vi "DAQ setting.vi"(8 "error in (no error)":errorcluster={"status"=TRUE, "code"=1026, "source"="Invoke Node in General Config.vi->Main Window.vi"}, 11 "vi reference":refnum<vi>) -> (0 "error Out":errorcluster={"status"=TRUE, "code"=1026, "source"="Invoke Node in General Config.vi->Main Window.vi"}, 3 "Out reference":refnum<vi>)   [LabVIEW 2015]
uses:
  Control Button/Exit.ctl
  Control Button/Save.ctl
  <vilib>/addons/database/Connection.llb/DB Tools Open Connec (String).vi
  <vilib>/addons/database/_DB Variant To Data/Database Variant To Data.xnode
  <vilib>/addons/database/NI_Database_API.lvlib
panel:
  out "error out":errorcluster={"status"=TRUE, "code"=97, "source"="NI_Database_API.lvlib:DB Tools Close Connection.vi->DAQ setting.vi<ERR>ADO Error: 0x00000061\r\nUnknown System Error in NI_Database_API.lvlib:DB Tools Close Connection.vi->DAQ setting.vi"}
  in  "read":bool=TRUE
  out "subarray":string[](array[string])=["PART CLAMPING CYL-1&2 SOL(P0.17)", "PART DECLAMPING CYL-1&2 SOL (P0.18)", "FLAP LOCKING CYL FDW SOL(P0.19)", "SCREWING UNIT UP SOL (P0.20)", "SCREWING UNIT DOWN SOL  (P0.21)", "Z DIRECTION CYL UP SOL Feeder Unit (P0.22)", "Z DIRECTION CYL Down SOL Feeder Unit (P0.23)", "SCREW PICKING CYL FWD Feeder Unit (P0.24)", "SCREW PICKING CYL REV Feeder Unit (P0.25)", "Demagneting Cyl UP SOL Feeder Unit (P0.26)", "Demagneting Cyl DOWN SOL Feeder Unit (P0.27)", "AIR ON SOL FOR FEEDER UNIT(P0.28)", "FIXTURE MOVING CYL FWD.(P0.29)", "FIXTURE MOVING CYL REV (P0.30", "LVDT UNIT UP SOL (P0.31)", "LVDT UNIT DOWN SOL (P1.0)", "DC NUT RUNNER START CMD (P1.1)", "DC NUT RUNNER RESET SIGNAL(P1.2)", "DC NUT RUNNER DIRECTION SIGNAL (P1.3)", "DC NUT RUNNER CYCLE-1 CMD (P1.4)", "DC NUT RUNNER CYCLE-2 CMD(P1.5)", "DC NUT RUNNER CYCLE-4 CMD (P1.6)", "TWL RED/FAULT WITH BUZZER (P1.7)", "TWL GREEN/OK (P2.0)", "TWL YELLOW/RUNNING (P2.1)", "Spare (P2.2)", "Spare (P2.3)", "Spare(P2.4)", "Spare (P2.5)", "Spare (P2.6)", "Spare (P2.7)", ""]
  in  "Save":T1=TRUE
  in  "Exit":T2
  in  "Tab Control":T3(tab)
  in  "DAQmx OutPut Setting":T4={"DAQmx OutPut_00"="Dev2/port0/line0", "DAQmx OutPut_01"="Dev2/port0/line1", "DAQmx OutPut_02"="Dev2/port0/line2", "DAQmx OutPut_03"="Dev2/port0/line3", "DAQmx OutPut_04"="Dev2/port0/line4", "DAQmx OutPut_05"="Dev2/port0/line5", "DAQmx OutPut_06"="Dev2/port0/line6", "DAQmx OutPut_07"="Dev2/port0/line7", "DAQmx OutPut_08"="Dev2/port0/line8", "DAQmx OutPut_09"="Dev2/port0/line9", "DAQmx OutPut_10"="Dev2/port0/line10", "DAQmx OutPut_11"="Dev2/port0/line11", "DAQmx OutPut_12"="Dev2/port0/line12", "DAQmx OutPut_13"="Dev2/port0/line13", "DAQmx OutPut_14"="Dev2/port0/line14", "DAQmx OutPut_15"="Dev2/port0/line15", "DAQmx OutPut_16"="Dev2/port1/line0", "DAQmx OutPut_17"="Dev2/port1/line1", "DAQmx OutPut_18"="Dev2/port1/line2", "DAQmx OutPut_19"="Dev2/port1/line3", "DAQmx OutPut_20"="Dev2/port1/line4", "DAQmx OutPut_21"="Dev2/port1/line5", "DAQmx OutPut_22"="Dev2/port1/line6", "DAQmx OutPut_23"="Dev2/port1/line7", "DAQmx OutPut_12 2"="Dev2/port2/line0", "DAQmx OutPut_13 2"="Dev2/port2/line1", "DAQmx OutPut_13 3"="Dev2/port2/line2", "DAQmx OutPut_13 4"="Dev2/port2/line3", "DAQmx OutPut_13 5"="Dev2/port2/line4", "DAQmx OutPut_13 6"="A", "String"="Dev1/port2/line2"}
  in  "DAQmx InPut Setting":T5={"DAQmx InPut_00"="Dev1/port0/line0", "DAQmx InPut_01"="Dev1/port0/line1", "DAQmx InPut_02"="Dev1/port0/line2", "DAQmx InPut_03"="Dev1/port0/line3", "DAQmx InPut_04"="Dev1/port0/line4", "DAQmx InPut_05"="Dev1/port0/line5", "DAQmx InPut_06"="Dev1/port0/line6", "DAQmx InPut_07"="Dev1/port0/line7", "DAQmx InPut_08"="Dev1/port1/line0", "DAQmx InPut_09"="Dev1/port1/line1", "DAQmx InPut_10"="Dev1/port1/line2", "DAQmx InPut_11"="Dev1/port1/line3", "DAQmx InPut_12"="Dev1/port1/line4", "DAQmx InPut_13"="Dev1/port1/line5", "DAQmx InPut_14"="Dev1/port1/line6", "DAQmx InPut_15"="Dev1/port1/line7", "Key"="A"}
  in  "DAQmx Analog Input Setting":T6={"DAQmx Analog Input_00"="Dev1/ai0", "DAQmx Analog Input_01"="Dev1/ai1", "DAQmx Analog Input_02"="Dev1/ai2", "DAQmx Analog Input_03"="Dev1/ai3", "DAQmx Analog Input_04"="Dev1/ai4", "DAQmx Analog Input_05"="Dev1/ai5", "DAQmx Analog Input_06"="Dev1/ai6", "DAQmx Analog Input_07"="Dev1/ai7", "DAQmx Analog Input_08"="Dev1/ai8", "DAQmx Analog Input_09"="Dev1/ai9", "DAQmx Analog Input_10"="Dev1/ai10", "DAQmx Analog Input_11"="Dev1/ai11", "DAQmx Analog Input_12"="Dev1/ai12", "DAQmx Analog Input_13"="Dev1/ai13", "DAQmx Analog Input_14"="Dev1/ai14", "DAQmx Analog Input_15"="Dev1/ai15", "DAQmx Analog Input_16"="Dev2/ai0", "DAQmx Analog Input_17"="Dev2/ai1", "DAQmx Analog Input_18"="Dev2/ai2", "DAQmx Analog Input_19"="Dev2/ai3", "DAQmx Analog Input_20"="Dev2/ai4", "DAQmx Analog Input_21"="Dev2/ai5", "DAQmx Analog Input_22"="Dev2/ai6", "DAQmx Analog Input_23"="Dev2/ai7", "DAQmx Analog Input_24"="Dev2/ai8", "DAQmx Analog Input_25"="Dev2/ai9", "DAQmx Analog Input_26"="Dev2/ai10", "DAQmx Analog Input_27"="Dev2/ai11", "DAQmx Analog Input_28"="Dev2/ai12", "DAQmx Analog Input_29"="Dev2/ai13", "DAQmx Analog Input_30"="Dev2/ai14", "DAQmx Analog Input_31"="Dev2/ai15", "String 2"="A"}
  in  "DAQmx  Counter In":tag
  in  "DAQmx  Counter In":tag
  in  "DAQmx Counter Out":tag
  # "Digital Output  Configuration"
  # "Digital Input Configuration"
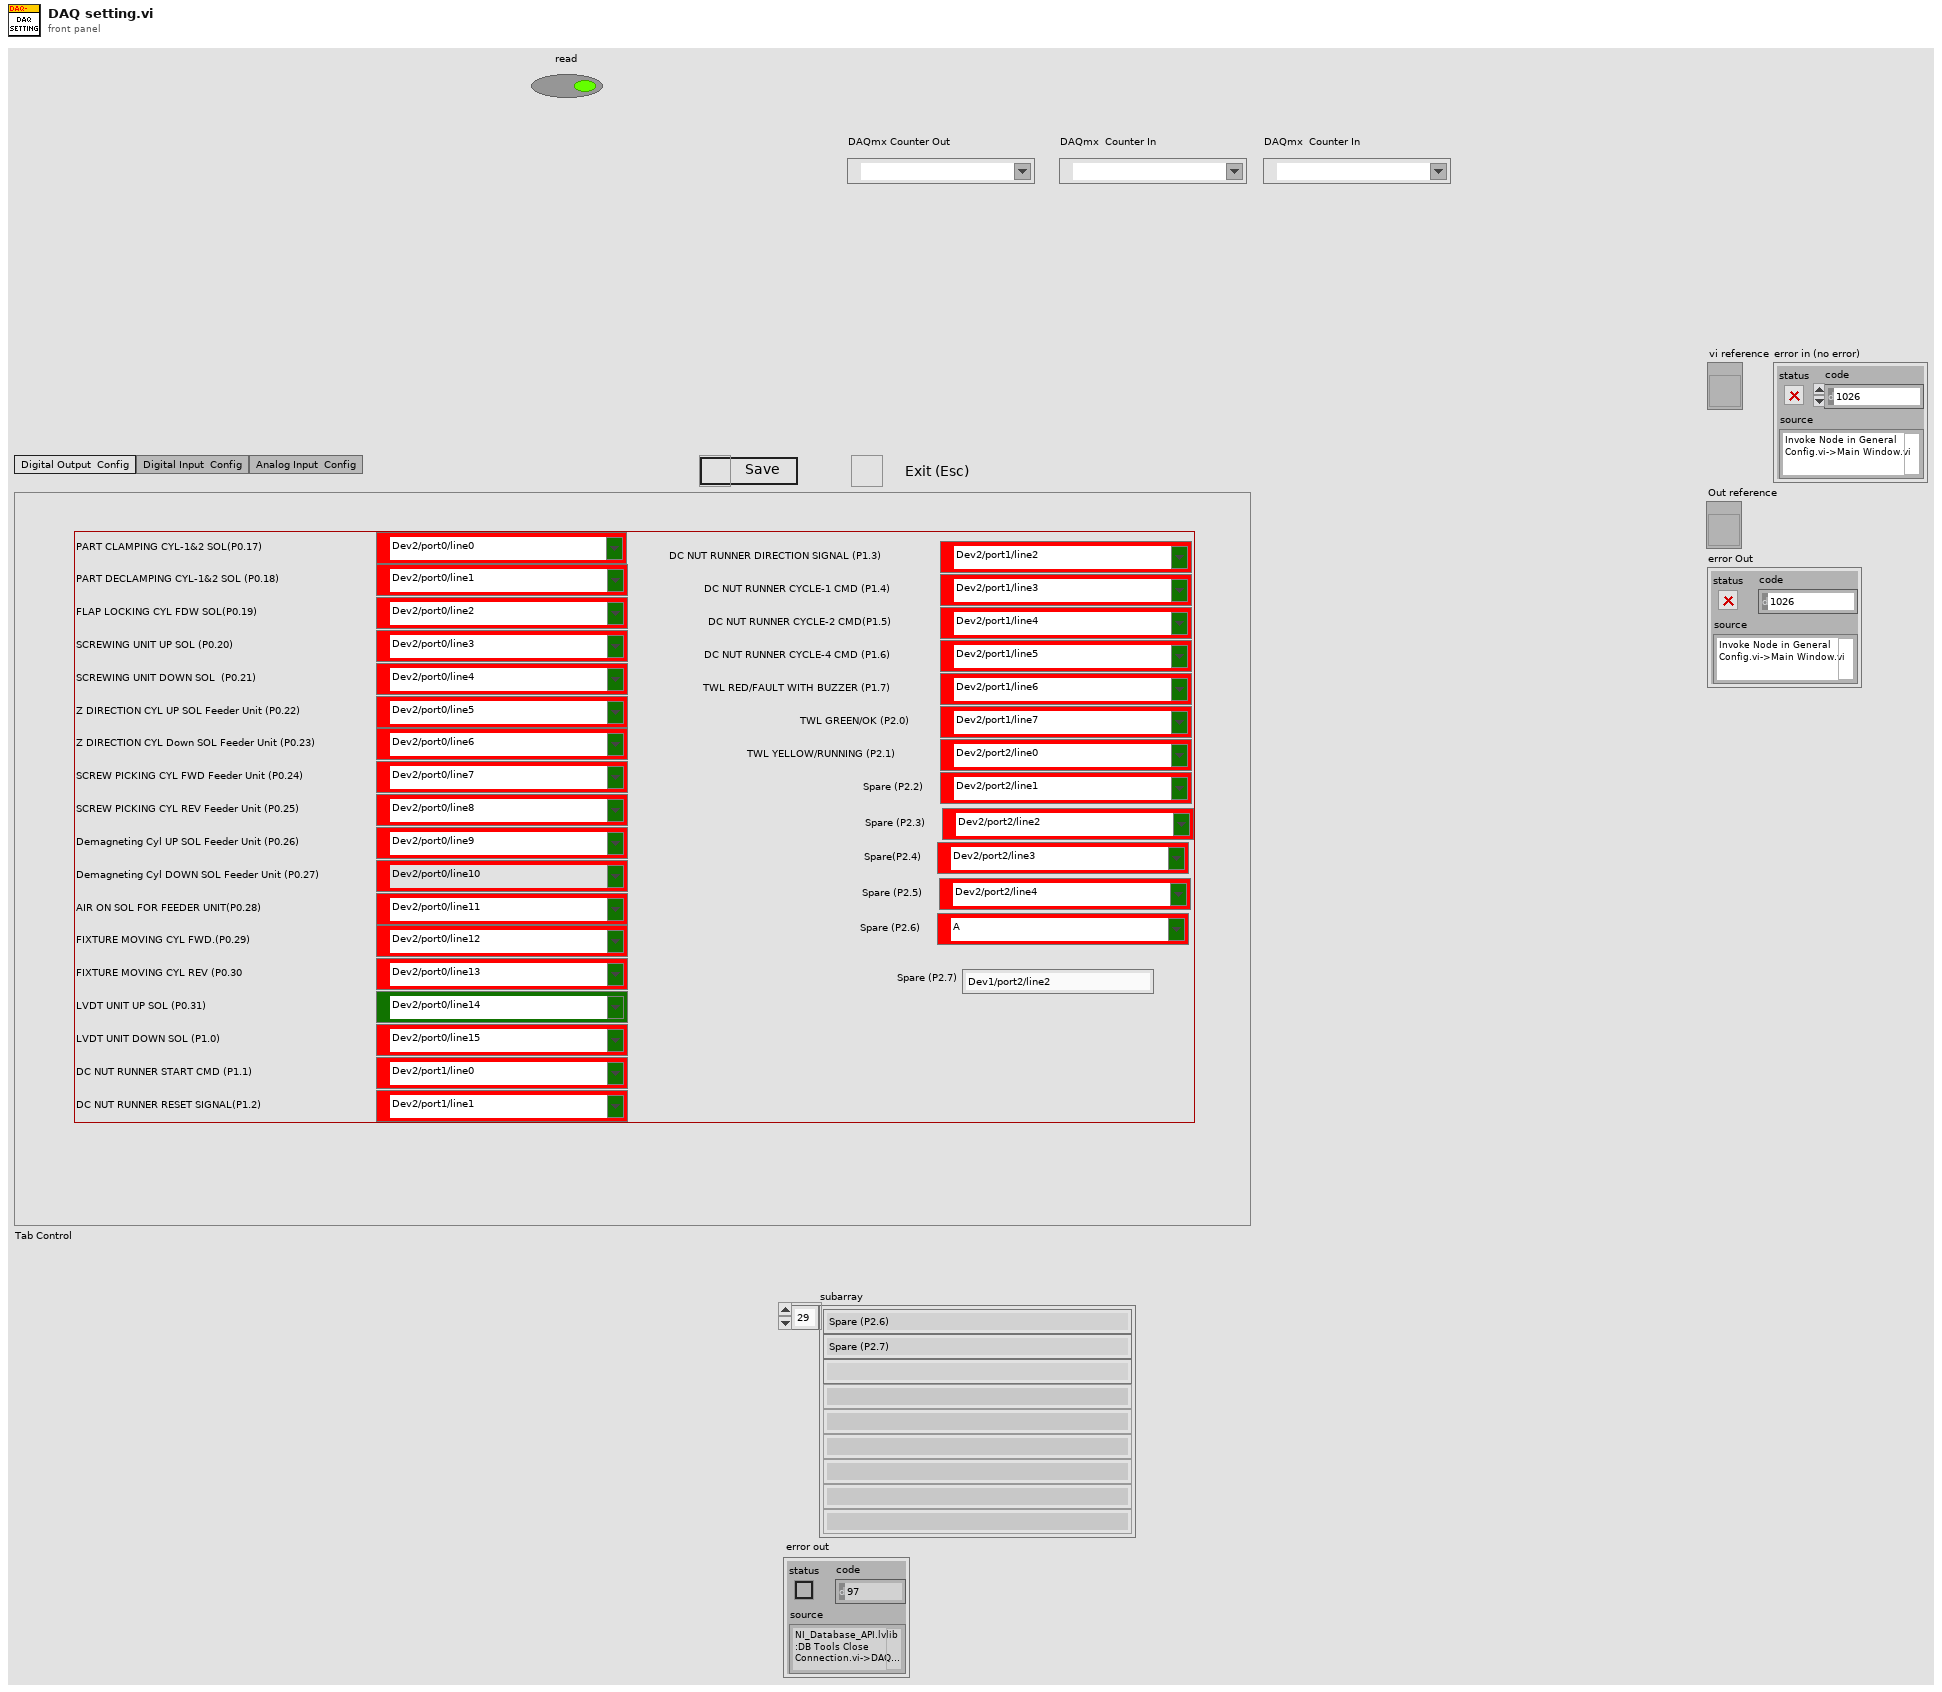
[diagram p1: front panel]
types:
  T1 = typedef "Save.ctl" = bool
  T2 = typedef "Exit.ctl" = bool
  T3 = enum32{"Digital Output  Config", "Digital Input  Config", "Analog Input  Config"}
  T4 = cluster{"DAQmx OutPut_00":tag, "DAQmx OutPut_01":tag, "DAQmx OutPut_02":tag, "DAQmx OutPut_03":tag, "DAQmx OutPut_04":tag, "DAQmx OutPut_05":tag, "DAQmx OutPut_06":tag, "DAQmx OutPut_07":tag, "DAQmx OutPut_08":tag, "DAQmx OutPut_09":tag, "DAQmx OutPut_10":tag, "DAQmx OutPut_11":tag, "DAQmx OutPut_12":tag, "DAQmx OutPut_13":tag, "DAQmx OutPut_14":tag, "DAQmx OutPut_15":tag, "DAQmx OutPut_16":tag, "DAQmx OutPut_17":tag, "DAQmx OutPut_18":tag, "DAQmx OutPut_19":tag, "DAQmx OutPut_20":tag, "DAQmx OutPut_21":tag, "DAQmx OutPut_22":tag, "DAQmx OutPut_23":tag, "DAQmx OutPut_12 2":tag, "DAQmx OutPut_13 2":tag, "DAQmx OutPut_13 3":tag, "DAQmx OutPut_13 4":tag, "DAQmx OutPut_13 5":tag, "DAQmx OutPut_13 6":tag, "String":string}
  T5 = cluster{"DAQmx InPut_00":tag, "DAQmx InPut_01":tag, "DAQmx InPut_02":tag, "DAQmx InPut_03":tag, "DAQmx InPut_04":tag, "DAQmx InPut_05":tag, "DAQmx InPut_06":tag, "DAQmx InPut_07":tag, "DAQmx InPut_08":tag, "DAQmx InPut_09":tag, "DAQmx InPut_10":tag, "DAQmx InPut_11":tag, "DAQmx InPut_12":tag, "DAQmx InPut_13":tag, "DAQmx InPut_14":tag, "DAQmx InPut_15":tag, "Key":string}
  T6 = cluster{"DAQmx Analog Input_00":tag, "DAQmx Analog Input_01":tag, "DAQmx Analog Input_02":tag, "DAQmx Analog Input_03":tag, "DAQmx Analog Input_04":tag, "DAQmx Analog Input_05":tag, "DAQmx Analog Input_06":tag, "DAQmx Analog Input_07":tag, "DAQmx Analog Input_08":tag, "DAQmx Analog Input_09":tag, "DAQmx Analog Input_10":tag, "DAQmx Analog Input_11":tag, "DAQmx Analog Input_12":tag, "DAQmx Analog Input_13":tag, "DAQmx Analog Input_14":tag, "DAQmx Analog Input_15":tag, "DAQmx Analog Input_16":tag, "DAQmx Analog Input_17":tag, "DAQmx Analog Input_18":tag, "DAQmx Analog Input_19":tag, "DAQmx Analog Input_20":tag, "DAQmx Analog Input_21":tag, "DAQmx Analog Input_22":tag, "DAQmx Analog Input_23":tag, "DAQmx Analog Input_24":tag, "DAQmx Analog Input_25":tag, "DAQmx Analog Input_26":tag, "DAQmx Analog Input_27":tag, "DAQmx Analog Input_28":tag, "DAQmx Analog Input_29":tag, "DAQmx Analog Input_30":tag, "DAQmx Analog Input_31":tag, "String 2":string}
  T7 = enum8{"Enabled", "Disabled", "Disabled and Grayed Out"}
  T8 = typedef "NI_Database_API.lvlib/Conn ObjectReference.ctl" = refnum<k1>
  T9 = cluster{"data[0]":string, "data[1]":string, "data[2]":string, "data[3]":string, "data[4]":string, "data[5]":string, "data[6]":string, "data[7]":string, "data[8]":string, "data[9]":string, "data[10]":string, "data[11]":string, "data[12]":string, "data[13]":string, "data[14]":string, "data[15]":string, "data[16]":string}
  T10 = cluster{"data[0]":string, "data[1]":string, "data[2]":string, "data[3]":string, "data[4]":string, "data[5]":string, "data[6]":string, "data[7]":string, "data[8]":string, "data[9]":string, "data[10]":string, "data[11]":string, "data[12]":string, "data[13]":string, "data[14]":string, "data[15]":string, "data[16]":string, "data[17]":string, "data[18]":string, "data[19]":string, "data[20]":string, "data[21]":string, "data[22]":string, "data[23]":string, "data[24]":string, "data[25]":string, "data[26]":string, "data[27]":string, "data[28]":string, "data[29]":string, "data[30]":string}
  T11 = cluster{"data[0]":string, "data[1]":string, "data[2]":string, "data[3]":string, "data[4]":string, "data[5]":string, "data[6]":string, "data[7]":string, "data[8]":string, "data[9]":string, "data[10]":string, "data[11]":string, "data[12]":string, "data[13]":string, "data[14]":string, "data[15]":string, "data[16]":string, "data[17]":string, "data[18]":string, "data[19]":string, "data[20]":string, "data[21]":string, "data[22]":string, "data[23]":string, "data[24]":string, "data[25]":string, "data[26]":string, "data[27]":string, "data[28]":string, "data[29]":string, "data[30]":string, "data[31]":string, "data[32]":string}
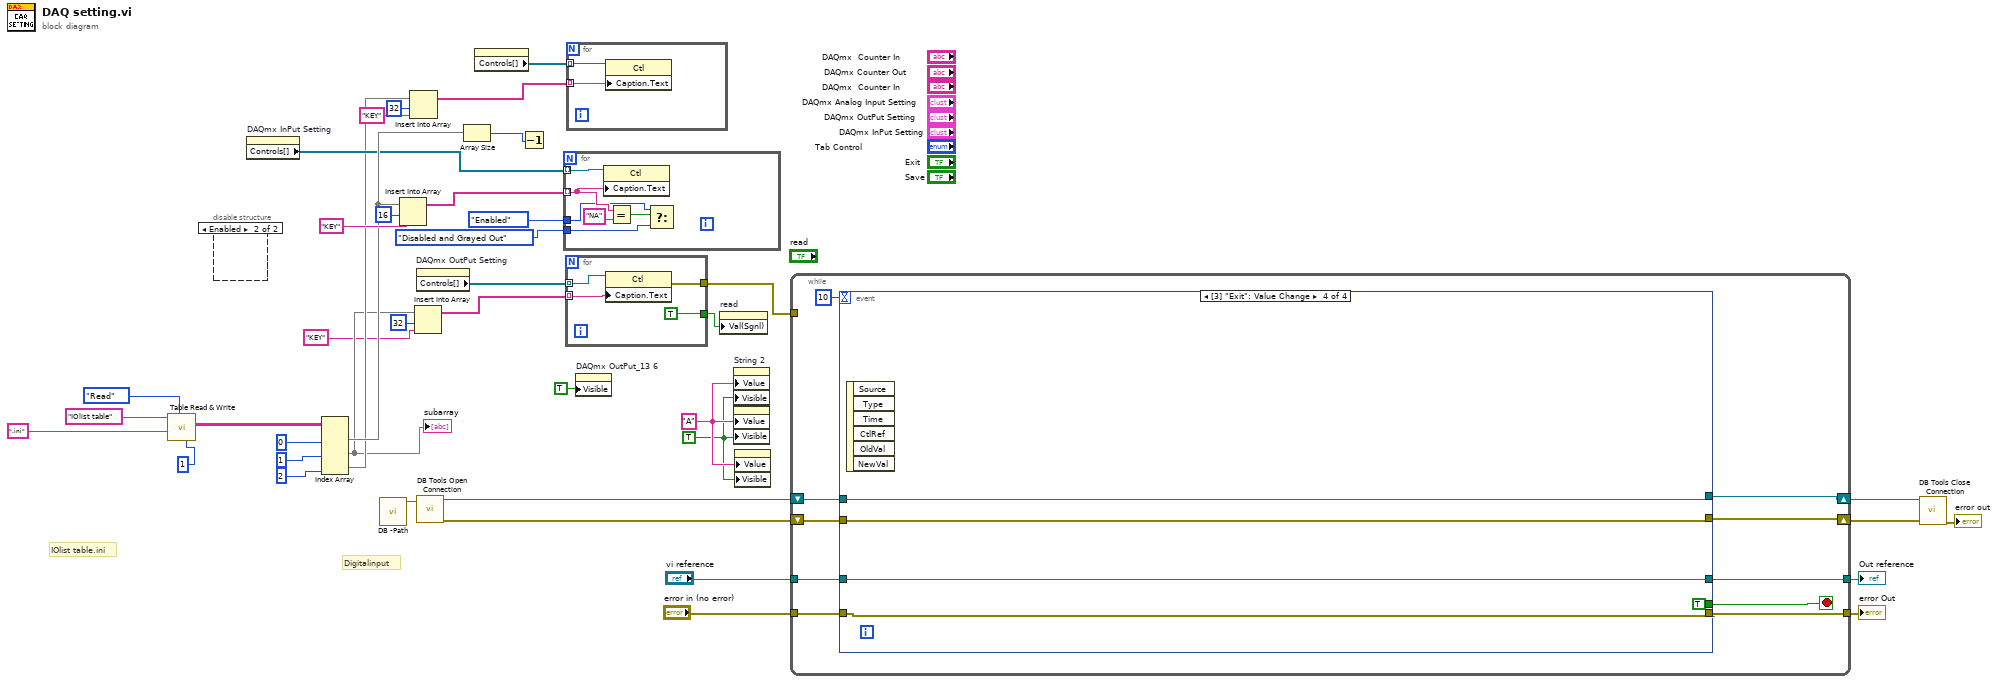
[diagram p0: block diagram]
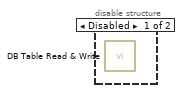
[diagram p2: hidden frame]
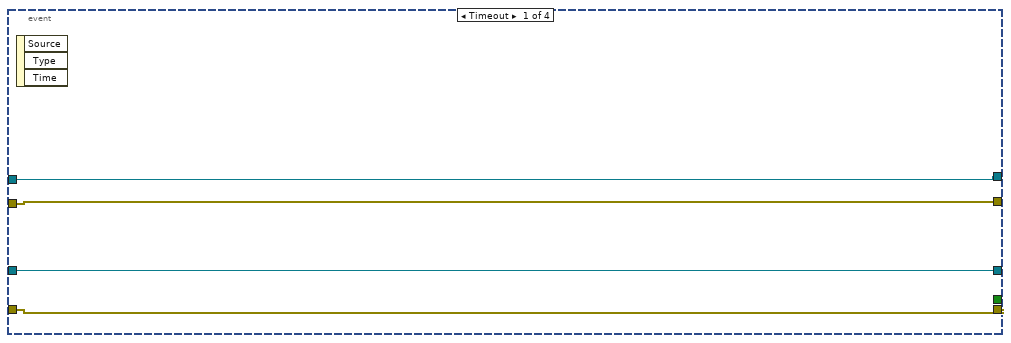
[diagram p3: hidden frame]
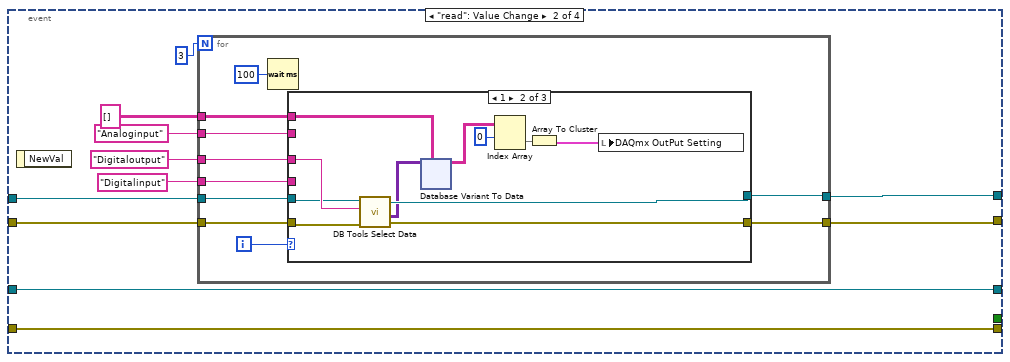
[diagram p4: hidden frame]
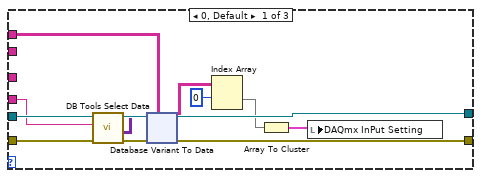
[diagram p5: hidden frame]
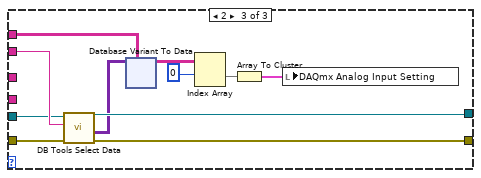
[diagram p6: hidden frame]
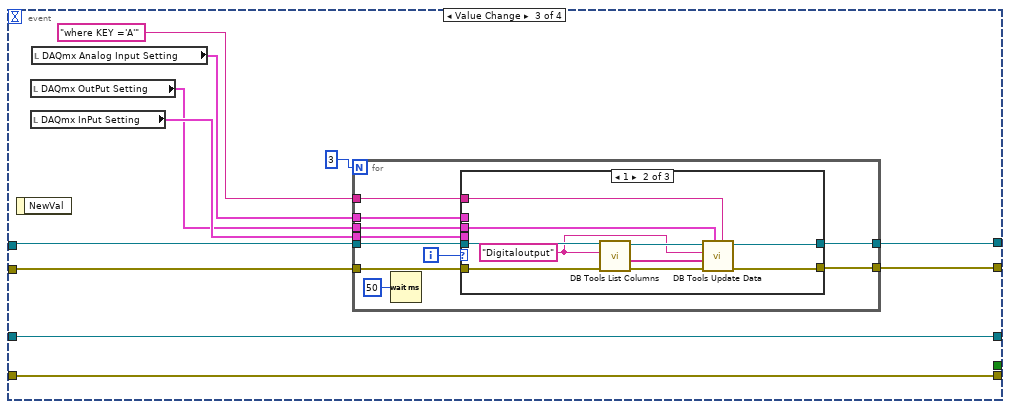
[diagram p7: hidden frame]
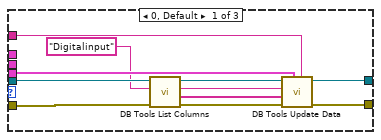
[diagram p8: hidden frame]
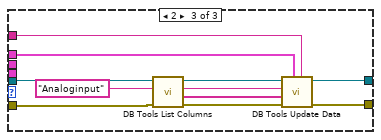
[diagram p9: hidden frame]
diagram:
  w2 = TRUE ("Visible")
  w3 = "A" ("Value")
  # "IOlist table.ini"
  # "Digitalinput"
  n1 = call "Table Read & Write.vi"("File Name"="IOlist table", "File type"=".ini", "Enum"=enum16{"Read", "Write"}."Read", "index"=1) -> ("Read Table"=w30:string[][])  [unwired: 5 in, 1 out]
  n2 = disable-structure shown="Enabled" {
    frame Disabled {
      n3 = call "DB Table Read & Write.vi"() -> ()  [unwired: 10 in, 2 out]
    }
    frame Enabled {
    }
  }
  n4 = property on="DAQmx InPut Setting" class="Clust (strict)"() -> ("Controls[]"=w13:refnum<vi>[])  [unwired: 2 in, 2 out]
  n5 = Index Array(array=w30, index (col) #1=0 ("disabled index (col)"), index (col) #2=1 ("index (col)"), index (col) #3=2 ("index (col)")) -> (element #1=w15:string[], element #2=w9:string[], element #3=w11:string[])  [unwired: 3 in]
  "subarray" <- w9
  n6 = call "DB -Path.vi"() -> ("String"=w27:string)  [unwired: 11 in]
  n7 = Insert Into Array(array=w15, index=16, new element="KEY" ("new element/subarray")) -> (w14:string[])
  n8 = Insert Into Array(array=w11, index=32, new element="KEY" ("new element/subarray")) -> (w4:string[])
  n9 = Insert Into Array(array=w9, index=32, new element="KEY" ("new element/subarray")) -> (w6:string[])
  n10 = property on="DAQmx OutPut Setting" class="Clust (strict)"() -> ("Controls[]"=w38:refnum<vi>[])  [unwired: 2 in, 2 out]
  n11 = call-poly <vilib>:"DB Tools Open Connection.vi"("connection information"=w27) -> ("error out"=w25:errorcluster, "connection reference"=w26:T8)  [unwired: 7 in]
  n12 = Array Size(array=w15) -> (size(s)=w18:i32)
  n13 = property on="DAQmx Analog Input Setting" class="Clust (strict)"() -> ("Controls[]"=w5:refnum<vi>[])  [unwired: 2 in, 2 out]
  n14 = Decrement(x=w18) -> ()  [unwired: 1 out]
  n15 = for {
    tunnel: w13 -> [w47] mode=indexing
    tunnel: w14 -> [w45] mode=indexing
    tunnel: T7."Enabled" ("Disabled") -> [w44]
    tunnel: T7."Disabled and Grayed Out" ("Disabled") -> [w43]
    n16 = property class="Ctl"(reference=w47, "Caption.Text"=w45) -> ()  [unwired: 1 in, 2 out]
    n17 = Equal?(x=w45, y="NA") -> (x = y?=w42:bool)
    n18 = Select(t=w44, s=w42, f=w43) -> ()  [unwired: 1 out]
  }
  n19 = for {
    tunnel: w38 -> [w51] mode=indexing
    tunnel: w6 -> [w50] mode=indexing
    tunnel: [w49] -> w29
    tunnel: [TRUE] -> w28
    n20 = property class="Ctl"(reference=w51, "Caption.Text"=w50) -> (error out=w49:errorcluster)  [unwired: 1 in, 1 out]
  }
  n21 = for {
    tunnel: w5 -> [w53] mode=indexing
    tunnel: w4 -> [w52] mode=indexing
    n22 = property class="Ctl"(reference=w53, "Caption.Text"=w52) -> ()  [unwired: 1 in, 2 out]
  }
  n23 = property on="DAQmx OutPut_13 6" class="DAQmxName"("Visible"=TRUE) -> ()  [unwired: 2 in, 2 out]
  n24 = property on="read" class="Bool (strict)"("Val(Sgnl)"=w28) -> ()  [unwired: 2 in, 2 out]
  n25 = property on="String 2" class="Str"("Value"=w3, "Visible"=w2) -> ()  [unwired: 2 in, 2 out]
  n26 = property on="Key" class="Str"("Value"=w3, "Visible"=w2) -> ()  [unwired: 2 in, 2 out]
  n27 = property on="String" class="Str"("Value"=w3, "Visible"=w2) -> ()  [unwired: 2 in, 2 out]
  n28 = while {
    tunnel: "vi reference" -> [w61]
    tunnel: "error in (no error)" -> [w60]
    tunnel: [w59] -> w35
    tunnel: [w58] -> w34
    tunnel: w29 -> [_]
    shift-right: [w55] -> w24
    shift-left: w26 -> [w57]
    shift-right: [w54] -> w23
    shift-left: w25 -> [w56]
    stop <- w62 stop-if-true
    n29 = event shown="[3] \"Exit\": Value Change" {
      selector: _ -> [_ _ _ _]
      dyn-events: _ -> [_ _ _ _]
      timeout: 10 -> [_ _ _ _]
      tunnel: [_ _ _ TRUE] -> w62
      tunnel: w61 -> [w67 w78 w265 w309]
      tunnel: w60 -> [w66 w77 w264 w308]
      tunnel: [w67 w78 w265 w309] -> w59
      tunnel: [w66 w77 w264 w308] -> w58
      tunnel: w57 -> [w65 w71 w263 w307]
      tunnel: w56 -> [w64 w70 w262 w306]
      tunnel: [w65 w73 w260 w307] -> w55
      tunnel: [w64 w72 w259 w306] -> w54
      event Timeout {
        n30 = event-data() -> ()  [unwired: 1 in, 3 out]
      }
      event "read": Value Change {
        n31 = event-data() -> ()  [unwired: 1 in, 1 out]
        n32 = for {
          N: 3 -> [_]
          tunnel: "Digitalinput" ("table") -> [w86]
          tunnel: w71 -> [w85]
          tunnel: w70 -> [w84]
          tunnel: [w83] -> w73
          tunnel: [w82] -> w72
          tunnel: "Digitaloutput" ("table") -> [w81]
          tunnel: "Analoginput" ("table") -> [w80]
          tunnel: string[][] [] -> [w79]
          i -> [w88]
          n33 = Wait (ms)(milliseconds to wait=u32 100) -> ()  [unwired: 1 out]
          n34 = case shown="1" w88 {
            tunnel: w86 -> [w94 _ _]
            tunnel: w85 -> [w99 w154 w207]
            tunnel: w84 -> [w98 w153 w206]
            tunnel: [w97 w151 w205] -> w83
            tunnel: [w96 w150 w204] -> w82
            tunnel: w81 -> [_ w155 _]
            tunnel: w80 -> [_ _ w209]
            tunnel: w79 -> [w95 w152 w208]
            frame 0, Default {
              n35 = call <vilib>:"DB Tools Select Data.vi"("error in (no error)"=w98, "table"=w94, "connection reference"=w99) -> ("error out"=w89:errorcluster, "data"=w93:variant[][], "connection reference out"=w97:T8)  [unwired: 3 in]
              n36 = xnode "Database Variant To Data"("database variant"=w93, "error in (no error)"=w89, "type"=w95) -> ("data"=w92:string[][], "error out"=w96:errorcluster)
              n37 = Index Array(array=w92, index (row)=0) -> (element=w91:string[])  [unwired: 1 in]
              n38 = Array To Cluster(array=w91) -> (cluster=w90:T9)
              n39 = local write "DAQmx InPut Setting"(w90) -> ()
            }
            frame 1 {
              n40 = call <vilib>:"DB Tools Select Data.vi"("error in (no error)"=w153, "table"=w155, "connection reference"=w154) -> ("error out"=w150:errorcluster, "data"=w149:variant[][], "connection reference out"=w151:T8)  [unwired: 3 in]
              n41 = xnode "Database Variant To Data"("database variant"=w149, "type"=w152) -> ("data"=w148:string[][])  [unwired: 1 in, 1 out]
              n42 = Index Array(array=w148, index (row)=0 ("disabled index (col)")) -> (element=w146:string[])  [unwired: 1 in]
              n43 = Array To Cluster(array=w146) -> (cluster=w145:T10)
              n44 = local write "DAQmx OutPut Setting"(w145) -> ()
            }
            frame 2 {
              n45 = call <vilib>:"DB Tools Select Data.vi"("error in (no error)"=w206, "table"=w209, "connection reference"=w207) -> ("error out"=w204:errorcluster, "data"=w202:variant[][], "connection reference out"=w205:T8)  [unwired: 3 in]
              n46 = xnode "Database Variant To Data"("database variant"=w202, "type"=w208) -> ("data"=w203:string[][])  [unwired: 1 in, 1 out]
              n47 = Index Array(array=w203, index (row)=0 ("disabled index (col)")) -> (element=w201:string[])  [unwired: 1 in]
              n48 = Array To Cluster(array=w201) -> (cluster=w200:T11)
              n49 = local write "DAQmx Analog Input Setting"(w200) -> ()
            }
          }
        }
      }
      event Value Change {
        n50 = event-data() -> ()  [unwired: 1 in, 1 out]
        n51 = local read "DAQmx OutPut Setting"() -> (w255:T4)
        n52 = local read "DAQmx InPut Setting"() -> (w261:T5)
        n53 = local read "DAQmx Analog Input Setting"() -> (w256:T6)
        n54 = for {
          N: 3 -> [_]
          tunnel: w263 -> [w274]
          tunnel: w262 -> [w273]
          tunnel: w256 -> [w272]
          tunnel: w255 -> [w271]
          tunnel: w261 -> [w270]
          tunnel: [w269] -> w260
          tunnel: [w268] -> w259
          tunnel: "where KEY ='A'" -> [w266]
          i -> [w275]
          n55 = Wait (ms)(milliseconds to wait=u32 50) -> ()  [unwired: 1 out]
          n56 = case shown="1" w275 {
            tunnel: w274 -> [w282 w291 w305]
            tunnel: w273 -> [w281 w292 w300]
            tunnel: w272 -> [_ _ w302]
            tunnel: w271 -> [_ w293 _]
            tunnel: w270 -> [w283 _ _]
            tunnel: [w285 w295 w304] -> w269
            tunnel: [w284 w294 w303] -> w268
            tunnel: w266 -> [w276 w286 w296]
            frame 0, Default {
              w277 = "Digitalinput" ("table")
              n57 = call <vilib>:"DB Tools List Columns.vi"("error in (no error)"=w281, "table"=w277, "connection reference"=w282) -> ("error out"=w278:errorcluster, "columns"=w280:string[], "connection reference out"=w279:T8)  [unwired: 1 in, 1 out]
              n58 = call <vilib>:"DB Tools Update Data.vi"("condition"=w276, "data"=w283, "error in (no error)"=w278, "columns"=w280, "table"=w277, "connection reference"=w279) -> ("error out"=w284:errorcluster, "connection reference out"=w285:T8)  [unwired: 4 in]
            }
            frame 1 {
              w287 = "Digitaloutput" ("table")
              n59 = call <vilib>:"DB Tools List Columns.vi"("error in (no error)"=w292, "table"=w287, "connection reference"=w291) -> ("error out"=w290:errorcluster, "columns"=w288:string[], "connection reference out"=w289:T8)  [unwired: 1 in, 1 out]
              n60 = call <vilib>:"DB Tools Update Data.vi"("condition"=w286, "data"=w293, "error in (no error)"=w290, "columns"=w288, "table"=w287, "connection reference"=w289) -> ("error out"=w294:errorcluster, "connection reference out"=w295:T8)  [unwired: 4 in]
            }
            frame 2 {
              w298 = "Analoginput" ("table")
              n61 = call <vilib>:"DB Tools List Columns.vi"("error in (no error)"=w300, "table"=w298, "connection reference"=w305) -> ("error out"=w299:errorcluster, "columns"=w297:string[], "connection reference out"=w301:T8)  [unwired: 1 in, 1 out]
              n62 = call <vilib>:"DB Tools Update Data.vi"("condition"=w296, "data"=w302, "error in (no error)"=w299, "columns"=w297, "table"=w298, "connection reference"=w301) -> ("error out"=w303:errorcluster, "connection reference out"=w304:T8)  [unwired: 4 in]
            }
          }
        }
      }
      event Value Change {
        n63 = event-data() -> ()  [unwired: 1 in, 6 out]
      }
    }
  }
  "Out reference" <- w35
  "error Out" <- w34
  n64 = call <vilib>:"DB Tools Close Connection.vi"("error in (no error)"=w23, "connection reference"=w24) -> ("error out"=→"error out":errorcluster)  [unwired: 5 in]
